vi "main.vi"() -> ()   [LabVIEW 2020]
doc: "该范例演示了通过VI查看其它VI的方法，还可运行和中止查看的VI。\n对于要中止的VI，应设置为可中止。对于无法中止的VI，可查看相关范例。"
uses:
  global/SettingVariable.vi
  global/GlobalVariable.vi
  utilities/TCPModbus_MasterClient.llb/MB Ethernet Master Query Read Input Registers (poly).vi
  utilities/TCPModbus_MasterClient.llb/MB Ethernet Master Query Write Multiple Registers (poly).vi
  <vilib>/Utility/config.llb/Write Key (Path).vi
  <vilib>/Utility/config.llb/NI_LVConfig.lvlib
panel:
  in  "退出":bool
  in  "Measure Square":bool
  in  "Physics Parameters Square":bool
  in  "Open Square":bool
  in  "Home Square":bool
  out "时间":string
  out "日期":string
  in  "MainPanel":enum32{"logo"}(tab)
  out "P2_8":dbl
  out "P2_7":dbl
  out "P2_6":dbl
  out "P2_5":dbl
  out "P2_4":dbl
  out "P2_3":dbl
  out "P2_2":dbl
  out "P2_1":dbl
  out "电流 2":dbl(slide)=1.0 scale=1e-13..0.0001 scale format="%#_2e"
  out "电流 1":dbl(slide)=1.0 scale=1e-13..0.0001 scale format="%#_2e"
  out "电压8":dbl(knob) caption="Gauge" scale=1.0..5.0
  out "电压7":dbl(knob)=1.0 caption="Gauge" scale=1.0..5.0
  out "电压6":dbl(knob)=1.0 caption="Gauge" scale=1.0..5.0
  out "电压5":dbl(knob)=1.0 caption="Gauge" scale=1.0..5.0
  out "电压4":dbl(knob)=1.0 caption="Gauge" scale=1.0..5.0
  out "电压3":dbl(knob)=1.0 caption="Gauge" scale=1.0..5.0
  out "电压2":dbl(knob) caption="Gauge" scale=1.0..5.0
  out "电压1":dbl(knob) caption="Gauge" scale=1.0..5.0
  in  "网络链接":bool
  # "iRho-100型反应性仪"
  # "Network"
  # "Current1"
  # "Current2"
  # "Voltage Output"
  # "Voltage Input"
  # "AC220V/50Hz"
  # "Ground"
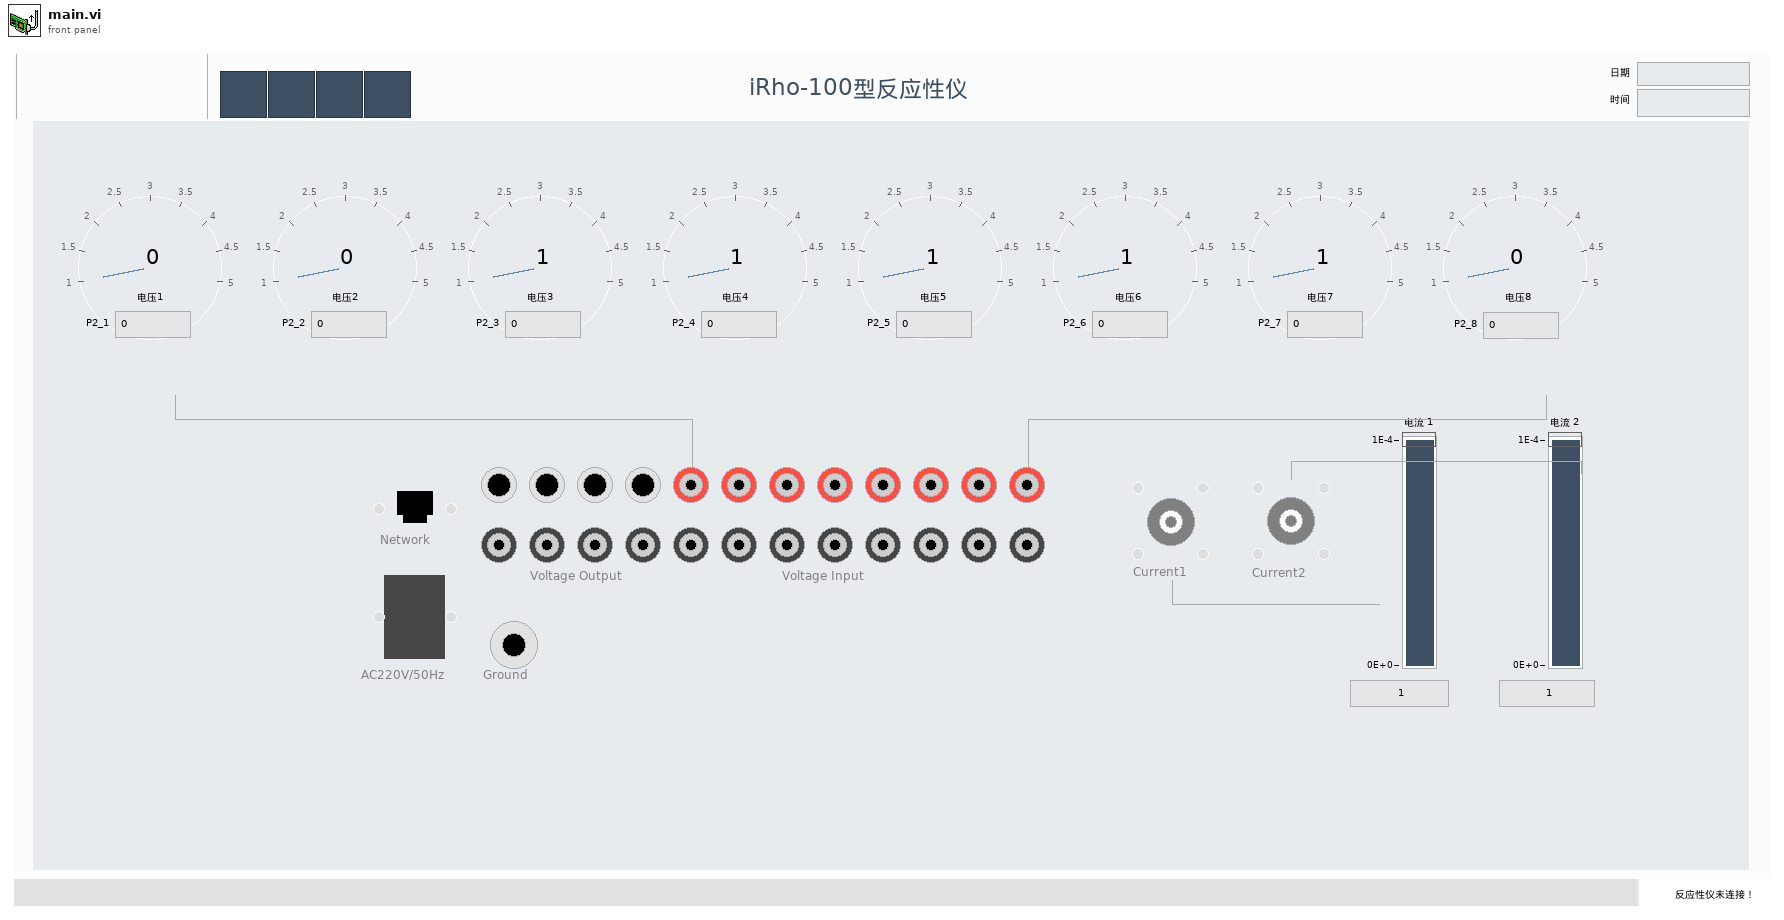
[diagram p1: front panel]
types:
  T1 = enum8{"Enabled", "Disabled", "Disabled and Grayed Out"}
  T2 = enum32{"Invalid", "Standard", "Closed", "Hidden", "Minimized", "Maximized"}
  T3 = cluster{"switch":bool, "name":string, "voltage upper":i32, "voltage lower":i32, "physics upper":dbl, "physics lower":dbl, "scale":u16}[]
  T4 = typedef "NI_LVConfig.lvlib/Config Data RefNum.ctl" = refnum<k1>
  T5 = enum32{"invalid app kind", "Development System", "Run Time System", "Student Edition", "Embedded LabVIEW", "Evaluation", "Custom"}
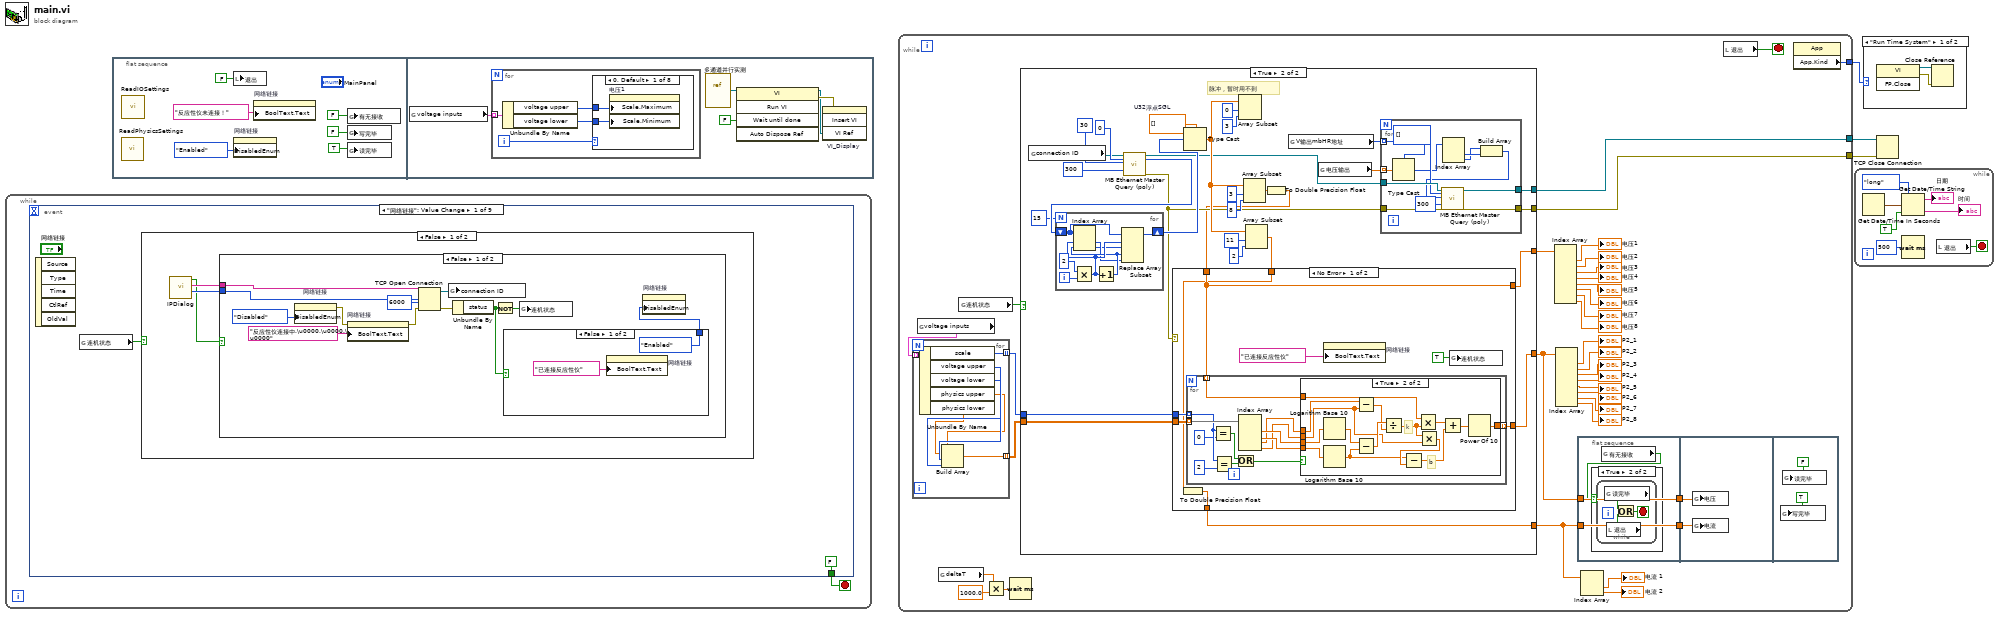
[diagram p0: block diagram]
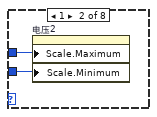
[diagram p2: hidden frame]
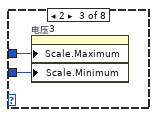
[diagram p3: hidden frame]
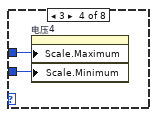
[diagram p4: hidden frame]
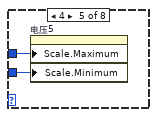
[diagram p5: hidden frame]
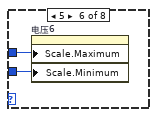
[diagram p6: hidden frame]
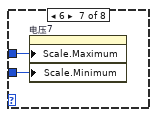
[diagram p7: hidden frame]
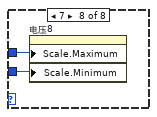
[diagram p8: hidden frame]
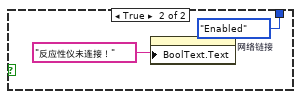
[diagram p9: hidden frame]
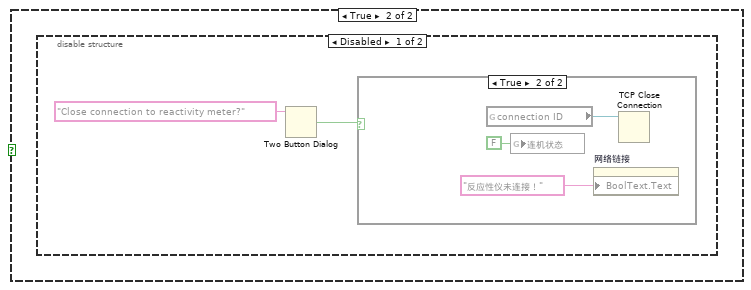
[diagram p11: hidden frame]
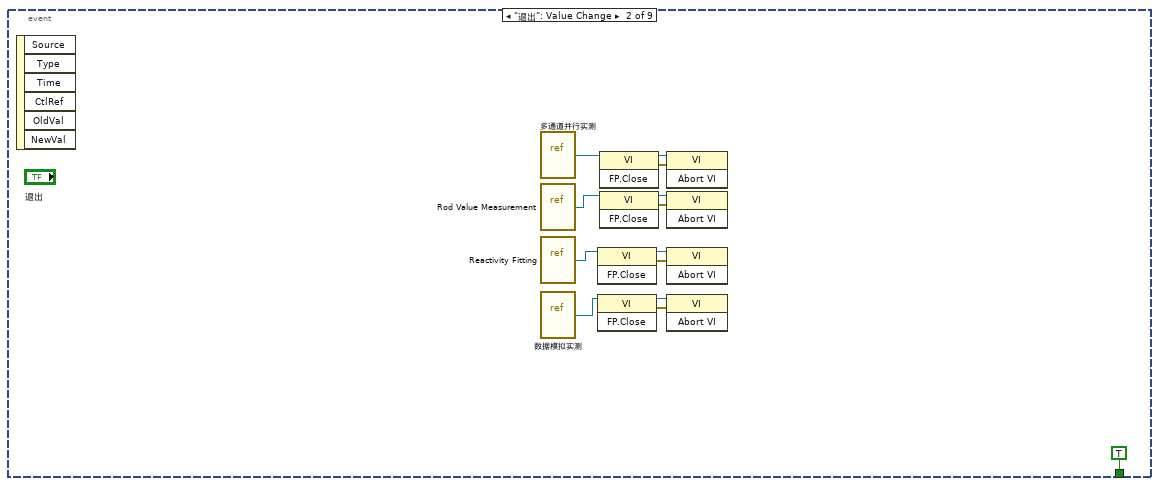
[diagram p14: hidden frame]
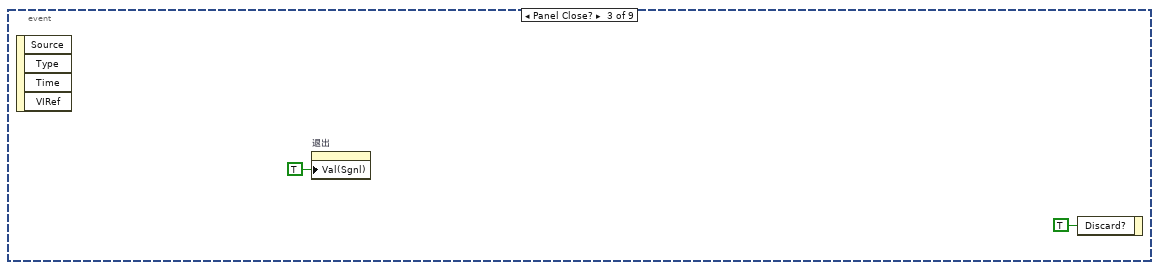
[diagram p15: hidden frame]
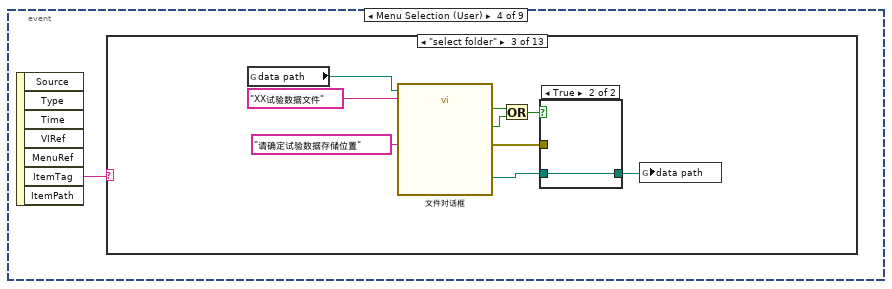
[diagram p16: hidden frame]
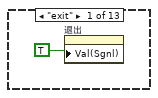
[diagram p17: hidden frame]
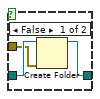
[diagram p19: hidden frame]
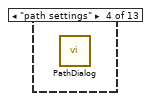
[diagram p20: hidden frame]
diagram:
  n1 = while {
    stop <- w4 stop-if-true
    n2 = event shown="[0] \"网络链接\": Value Change" {
      selector: _ -> [_ _ _ _ _ _ _ _ _]
      dyn-events: _ -> [_ _ _ _ _ _ _ _ _]
      timeout: _ -> [_ _ _ _ _ _ _ _ _]
      tunnel: [FALSE TRUE _ _ _ _ _ _ _] -> w4
      event "网络链接": Value Change {
        n3 = event-data() -> ()  [unwired: 1 in, 5 out]
        n4 = global read "GlobalVariable.vi" "连机状态"() -> (w5:bool)
        n5 = case shown="False" w5 {
          frame False {
            n6 = call "IPDialog.vi"() -> ("port"=w9:u16, "IP"=w8:string, "Cancelled?"=w7:bool)  [unwired: 9 in]
            n7 = case shown="False" w7 {
              tunnel: w9 -> [w12 _]
              tunnel: w8 -> [w11 _]
              frame False {
                n8 = property on="网络链接" class="Bool"("DisabledEnum"=T1."Disabled" ("Disabled")) -> (error out=w15:errorcluster)  [unwired: 2 in, 1 out]
                n9 = property on="网络链接" class="Bool"(error in=w15, "BoolText.Text"="反应性仪连接中.\u0000.\u0000.\u0000") -> (error out=w18:errorcluster)  [unwired: 1 in, 1 out]
                n10 = TCP Open Connection(address=w11, remote port or service name=w12, timeout ms (60000)=6000, error in (no error)=w18) -> (connection ID=w17:refnum<k5>, error out=w13:errorcluster)  [unwired: 1 out]
                n11 = global write "GlobalVariable.vi" "connection ID"(w17) -> ()
                n12 = Unbundle By Name(w13) -> ("status"=w19:bool)
                n13 = Not(x=w19) -> (.not. x?=w20:bool)
                n14 = case shown="False" w19 {
                  tunnel: [T1."Enabled" ("Disabled") T1."Enabled" ("Disabled")] -> w10
                  frame False {
                    n15 = property on="网络链接" class="Bool"("BoolText.Text"="已连接反应性仪") -> ()  [unwired: 2 in, 2 out]
                  }
                  frame True {
                    n16 = property on="网络链接" class="Bool"("BoolText.Text"="反应性仪未连接！") -> ()  [unwired: 2 in, 2 out]
                  }
                }
                n17 = global write "GlobalVariable.vi" "连机状态"(w20) -> ()
                n18 = property on="网络链接" class="Bool"("DisabledEnum"=w10) -> ()  [unwired: 2 in, 2 out]
              }
              frame True {
              }
            }
          }
          frame True {
            n19 = disable-structure shown="Disabled" {
              frame Disabled {
                n20 = Two Button Dialog(message="Close connection to reactivity meter?") -> (T button?=w26:bool)  [unwired: 2 in]
                n21 = case shown="True" w26 {
                  frame False {
                  }
                  frame True {
                    n22 = global read "GlobalVariable.vi" "connection ID"() -> (w30:refnum<k5>)
                    n23 = global write "GlobalVariable.vi" "连机状态"(FALSE ("连机状态")) -> ()
                    n24 = property on="网络链接" class="Bool"("BoolText.Text"="反应性仪未连接！" ("Boolean Text.Text")) -> ()  [unwired: 2 in, 2 out]
                    n25 = TCP Close Connection ("关闭TCP连接")(connection ID=w30) -> ()  [unwired: 1 in, 3 out]
                  }
                }
              }
              frame Enabled {
              }
            }
          }
        }
      }
      event "退出": Value Change {
        n26 = event-data() -> ()  [unwired: 1 in, 6 out]
        n27 = vi-ref "多通道并行实测.vi"() -> (w42:refnum<vi>)
        n28 = vi-ref "Rod Value Measurement.vi"() -> (w41:refnum<vi>)
        n29 = vi-ref "Reactivity Fitting.vi"() -> (w39:refnum<vi>)
        n30 = vi-ref "数据模拟实测.vi"() -> (w40:refnum<vi>)
        n31 = invoke class="VI" method="FP.Close"(reference=w39) -> (reference out=w34:refnum<vi>, error out=w33:errorcluster)  [unwired: 2 in, 1 out]
        n32 = invoke class="VI" method="FP.Close"(reference=w40) -> (reference out=w32:refnum<vi>, error out=w31:errorcluster)  [unwired: 2 in, 1 out]
        n33 = invoke class="VI" method="FP.Close"(reference=w42) -> (reference out=w38:refnum<vi>, error out=w37:errorcluster)  [unwired: 2 in, 1 out]
        n34 = invoke class="VI" method="FP.Close"(reference=w41) -> (reference out=w36:refnum<vi>, error out=w35:errorcluster)  [unwired: 2 in, 1 out]
        n35 = invoke class="VI" method="Abort VI"(reference=w38, error in=w37) -> ()  [unwired: 1 in, 3 out]
        n36 = invoke class="VI" method="Abort VI"(reference=w36, error in=w35) -> ()  [unwired: 1 in, 3 out]
        n37 = invoke class="VI" method="Abort VI"(reference=w34, error in=w33) -> ()  [unwired: 1 in, 3 out]
        n38 = invoke class="VI" method="Abort VI"(reference=w32, error in=w31) -> ()  [unwired: 1 in, 3 out]
      }
      event Panel Close? {
        n39 = event-data() -> ()  [unwired: 1 in, 4 out]
        n40 = property on="退出" class="Bool (strict)"("Val(Sgnl)"=TRUE ("Value (Signaling)")) -> ()  [unwired: 2 in, 2 out]
        n41 = event-data("Discard?"=TRUE) -> ()  [unwired: 1 in, 1 out]
      }
      event Menu Selection (User) {
        n42 = event-data() -> ("ItemTag"=w46:string)  [unwired: 1 in, 6 out]
        n43 = case shown="\"select folder\"" w46 {
          frame "exit" {
            n44 = property on="退出" class="Bool (strict)"("Val(Sgnl)"=TRUE) -> ()  [unwired: 2 in, 2 out]
          }
          frame Default {
          }
          frame "select folder" {
            n45 = global read "SettingVariable.vi" "data path"() -> (w49:path)
            n46 = call "文件对话框"("start path"=w49, "prompt"="请确定试验数据存储位置", "default name"="XX试验数据文件") -> ("selected path"=w56:path, "exists"=w54:bool, "cancelled"=w52:bool, "error out"=w55:errorcluster)  [unwired: 9 in]
            n47 = Or(x=w54, y=w52) -> (x .or. y?=w53:bool)
            n48 = case shown="True" w53 {
              tunnel: w56 -> [w59 w60]
              tunnel: w55 -> [w58 _]
              tunnel: [w57 w60] -> w48
              frame False {
                n49 = Create Folder(path (use dialog)=w59, error in=w58) -> (created path=w57:path)  [unwired: 1 in, 2 out]
              }
              frame True {
              }
            }
            n50 = global write "SettingVariable.vi" "data path"(w48) -> ()
          }
          frame "path settings" {
            n51 = call "PathDialog.vi"() -> ()  [unwired: 11 in, 1 out]
          }
          frame "physics settings" {
            n52 = call "PhysicsDialog.vi"() -> ()  [unwired: 1 in]
          }
          frame "input settings" {
            n53 = call "InputDialog.vi"() -> ("Cancelled?"=w61:bool)  [unwired: 9 in]
            n54 = case shown="True" w61 {
              frame False {
              }
              frame True {
                n55 = global read "SettingVariable.vi" "voltage inputs"() -> (w62:T3)
                n56 = for {
                  tunnel: w62 -> [w66] mode=indexing
                  i -> [w65]
                  n57 = Unbundle By Name(w66) -> ("voltage upper"=w64:i32, "voltage lower"=w63:i32)
                  n58 = case shown="0, Default" w65 {
                    tunnel: w64 -> [w68 w70 w72 w74 w76 w78 w80 w82]
                    tunnel: w63 -> [w67 w69 w71 w73 w75 w77 w79 w81]
                    frame 0, Default {
                      n59 = property on="电压1" class="Knob (strict)"("Scale.Maximum"=w68, "Scale.Minimum"=w67) -> ()  [unwired: 2 in, 2 out]
                    }
                    frame 1 {
                      n60 = property on="电压2" class="Knob (strict)"("Scale.Maximum"=w70, "Scale.Minimum"=w69) -> ()  [unwired: 2 in, 2 out]
                    }
                    frame 2 {
                      n61 = property on="电压3" class="Knob (strict)"("Scale.Maximum"=w72, "Scale.Minimum"=w71) -> ()  [unwired: 2 in, 2 out]
                    }
                    frame 3 {
                      n62 = property on="电压4" class="Knob (strict)"("Scale.Maximum"=w74, "Scale.Minimum"=w73) -> ()  [unwired: 2 in, 2 out]
                    }
                    frame 4 {
                      n63 = property on="电压5" class="Knob (strict)"("Scale.Maximum"=w76, "Scale.Minimum"=w75) -> ()  [unwired: 2 in, 2 out]
                    }
                    frame 5 {
                      n64 = property on="电压6" class="Knob (strict)"("Scale.Maximum"=w78, "Scale.Minimum"=w77) -> ()  [unwired: 2 in, 2 out]
                    }
                    frame 6 {
                      n65 = property on="电压7" class="Knob (strict)"("Scale.Maximum"=w80, "Scale.Minimum"=w79) -> ()  [unwired: 2 in, 2 out]
                    }
                    frame 7 {
                      n66 = property on="电压8" class="Knob (strict)"("Scale.Maximum"=w82, "Scale.Minimum"=w81) -> ()  [unwired: 2 in, 2 out]
                    }
                  }
                }
              }
            }
          }
          frame "output settings" {
            n67 = call "OutputDialog.vi"() -> ()  [unwired: 11 in, 1 out]
          }
          frame "homepage" {
            n68 = property on="VI_Display" class="SubPnl"("Visible"=FALSE) -> ()  [unwired: 2 in, 2 out]
          }
          frame "monitor" {
            n69 = property on="VI_Display" class="SubPnl"("Visible"=TRUE) -> ()  [unwired: 2 in, 2 out]
          }
          frame "rod measurement" {
            n70 = vi-ref "Rod Value Measurement.vi"() -> (w87:refnum<vi>)
            n71 = invoke class="VI" method="FP.Open"(reference=w87, "Activate"=TRUE ("Activate?"), "State"=T2."Standard") -> (reference out=w88:refnum<vi>)  [unwired: 2 in, 4 out]
            n72 = invoke class="VI" method="Run VI"(reference=w88, "Wait until done"=FALSE ("Wait Until Done"), "Auto Dispose Ref"=FALSE ("Auto Dispose Reference")) -> ()  [unwired: 2 in, 5 out]
          }
          frame "reactivity fitting" {
            n73 = vi-ref "Reactivity Fitting.vi"() -> (w93:refnum<vi>)
            n74 = invoke class="VI" method="FP.Open"(reference=w93, "Activate"=TRUE ("Activate?"), "State"=T2."Standard") -> (reference out=w94:refnum<vi>)  [unwired: 2 in, 4 out]
            n75 = invoke class="VI" method="Run VI"(reference=w94, "Wait until done"=FALSE ("Wait Until Done"), "Auto Dispose Ref"=FALSE ("Auto Dispose Reference")) -> ()  [unwired: 2 in, 5 out]
          }
          frame "history simulation" {
            n76 = vi-ref "数据模拟实测.vi"() -> (w99:refnum<vi>)
            n77 = invoke class="VI" method="FP.Open"(reference=w99, "Activate"=TRUE ("Activate?"), "State"=T2."Standard") -> (reference out=w100:refnum<vi>)  [unwired: 2 in, 4 out]
            n78 = invoke class="VI" method="Run VI"(reference=w100, "Wait until done"=FALSE ("Wait Until Done"), "Auto Dispose Ref"=FALSE ("Auto Dispose Reference")) -> ()  [unwired: 2 in, 5 out]
          }
          frame "about" {
            n79 = call "About.vi"() -> ()  [unwired: 1 in]
          }
        }
      }
      event "Home Square": Value Change {
        n80 = event-data() -> ()  [unwired: 1 in, 6 out]
        n81 = property on="VI_Display" class="SubPnl"("Visible"=FALSE) -> ()  [unwired: 2 in, 2 out]
      }
      event "Measure Square": Value Change {
        n82 = event-data() -> ()  [unwired: 1 in, 6 out]
        n83 = property on="VI_Display" class="SubPnl"("Visible"=TRUE) -> ()  [unwired: 2 in, 2 out]
      }
      event "Open Square": Value Change {
        n84 = event-data() -> ()  [unwired: 1 in, 6 out]
        n85 = global read "SettingVariable.vi" "data path"() -> (w105:path)
        n86 = call <vilib>:"Space Constant.vi"() -> ("String"=w119:string)
        n87 = Path To String(path=w105) -> (string=w116:string)
        n88 = Concatenate Strings("explorer" ("字符串"), w119, w116) -> (w117:string)
        n89 = call <vilib>:"System Exec.vi"("command line"=w117) -> ()  [unwired: 7 in, 4 out]
        n90 = call <vilib>:"Application Directory.vi"() -> ("Application Directory"=w111:path)
        n91 = Build Path(base path=w111, name or relative path=path "configure.ini") -> (appended path=w112:path)
        n92 = call <vilib>:"Open Config Data.vi"("configuration file path"=w112) -> ("error out"=w114:errorcluster, "refnum"=w113:T4)  [unwired: 2 in, 7 out]
        n93 = call-poly <vilib>:"Write Key.vi"("section"="Path", "error in (no error)"=w114, "value"=w105, "key"="data" ("section"), "refnum"=w113) -> ("error out"=w109:errorcluster, "refnum out"=w110:T4)  [unwired: 4 in, 1 out]
        n94 = call <vilib>:"Close Config Data.vi"("error in (no error)"=w109, "refnum"=w110) -> ("error out"=w115:errorcluster)  [unwired: 1 in, 8 out]
        n95 = call <vilib>:"Simple Error Handler.vi"("error in (no error)"=w115) -> ()  [unwired: 1 in, 8 out]
      }
      event "Physics Parameters Square": Value Change {
        n96 = event-data() -> ()  [unwired: 1 in, 6 out]
        n97 = call "PhysicsDialog.vi"() -> ()  [unwired: 1 in]
      }
      event "时间": Shortcut Menu Selection (User) {
        n98 = event-data() -> ("ItemTag"=w120:string)  [unwired: 1 in, 7 out]
        n99 = case shown="\"time calibration\", Default" w120 {
          frame "time calibration", Default {
            n100 = global read "GlobalVariable.vi" "连机状态"() -> (w121:bool)
            n101 = case shown="True" w121 {
              frame False {
                n102 = One Button Dialog(message="未连接反应性仪") -> ()  [unwired: 1 in, 1 out]
              }
              frame True {
                w129 = "%x" ("格式字符串")
                w130 = u16[] [] ("数组类型(2D Dbl)")
                n103 = Get Date/Time String(want seconds? (F)=TRUE ("需要秒？(F)")) -> (date string=w146:string, time string=w145:string)  [unwired: 2 in]
                n104 = Spreadsheet String To Array(delimiter (Tab)="/" ("分隔符(Tab)"), format string=w129, spreadsheet string=w146, array type (2D Dbl)=w130) -> (array=w142:u16[])
                n105 = Spreadsheet String To Array(delimiter (Tab)=":" ("分隔符(Tab)"), format string=w129, spreadsheet string=w145, array type (2D Dbl)=w130) -> (array=w140:u16[])
                n106 = Index Array(array=w142, index=0 ("索引")) -> (element=w144:u16)
                n107 = Subtract(x=w144, y=u16 8192) -> (x-y=w143:u16)
                n108 = Replace Array Subset(array=w142, new element=w143, index=0 ("索引")) -> (w141:u16[])
                n109 = Build Array (concatenate)(w141, w140) -> (w139:u16[])
                n110 = To Unsigned Byte Integer(number=w139) -> (unsigned 8bit integer=w138:u8[])
                n111 = for {
                  N: 3 -> [_]
                  shift-right: [w148] -> w137
                  shift-left: w138 -> [w153]
                  i -> [w155]
                  n112 = Multiply(x=2, y=w155) -> (x*y=w152:i32)
                  n113 = Increment(x=w152) -> (x+1=w151:i32)
                  n114 = Index Array(array=w153, index #1=w152, index #2=w151) -> (element #1=w150:u8, element #2=w149:u8)
                  n115 = Replace Array Subset(array=w153, new element #1=w149, index #1=w152, new element #2=w150, index #2=w151) -> (w148:u8[])
                }
                n116 = global read "GlobalVariable.vi" "connection ID"() -> (w123:refnum<k5>)
                n117 = Type Cast(type=u16[] [] ("Input Registers"), x=w137) -> (*(type *) &x=w125:u16[])
                n118 = call-poly "MB Ethernet Master Query (poly).vi"("TCP Connection Refnum in"=w123, "Starting Address"=u16 65436, "Registers"=w125) -> ("error out"=w124:errorcluster)  [unwired: 3 in, 13 out]
                n119 = case shown="Error .." w124 {
                  frame No Error {
                  }
                  frame Error {
                    n120 = One Button Dialog(message="写入失败！请检查网络连接。") -> ()  [unwired: 1 in, 1 out]
                  }
                }
              }
            }
          }
        }
      }
    }
  }
  n121 = flat-sequence {
    frame #0 {
      n122 = call "ReadPhysicsSettings.vi"() -> ()  [unwired: 12 in]
      n123 = call "ReadIOSettings.vi"() -> ()  [unwired: 12 in]
      n124 = local write "退出"(FALSE ("退出")) -> ()
      n125 = property on="网络链接" class="Bool"("DisabledEnum"=T1."Enabled" ("Disabled")) -> ()  [unwired: 2 in, 2 out]
      n126 = property on="网络链接" class="Bool"("BoolText.Text"="反应性仪未连接！") -> ()  [unwired: 2 in, 2 out]
      n127 = global write "GlobalVariable.vi" "有无接收"(FALSE ("读完毕")) -> ()
      n128 = global write "GlobalVariable.vi" "写完毕"(FALSE ("读完毕")) -> ()
      n129 = global write "GlobalVariable.vi" "读完毕"(TRUE ("读完毕")) -> ()
    }
    frame #1 {
      n130 = global read "SettingVariable.vi" "voltage inputs"() -> (w166:T3)
      n131 = for {
        tunnel: w166 -> [w170] mode=indexing
        i -> [w169]
        n132 = Unbundle By Name(w170) -> ("voltage upper"=w168:i32, "voltage lower"=w167:i32)
        n133 = case shown="0, Default" w169 {
          tunnel: w168 -> [w172 w174 w176 w178 w180 w182 w184 w186]
          tunnel: w167 -> [w171 w173 w175 w177 w179 w181 w183 w185]
          frame 0, Default {
            n134 = property on="电压1" class="Knob (strict)"("Scale.Maximum"=w172, "Scale.Minimum"=w171) -> ()  [unwired: 2 in, 2 out]
          }
          frame 1 {
            n135 = property on="电压2" class="Knob (strict)"("Scale.Maximum"=w174, "Scale.Minimum"=w173) -> ()  [unwired: 2 in, 2 out]
          }
          frame 2 {
            n136 = property on="电压3" class="Knob (strict)"("Scale.Maximum"=w176, "Scale.Minimum"=w175) -> ()  [unwired: 2 in, 2 out]
          }
          frame 3 {
            n137 = property on="电压4" class="Knob (strict)"("Scale.Maximum"=w178, "Scale.Minimum"=w177) -> ()  [unwired: 2 in, 2 out]
          }
          frame 4 {
            n138 = property on="电压5" class="Knob (strict)"("Scale.Maximum"=w180, "Scale.Minimum"=w179) -> ()  [unwired: 2 in, 2 out]
          }
          frame 5 {
            n139 = property on="电压6" class="Knob (strict)"("Scale.Maximum"=w182, "Scale.Minimum"=w181) -> ()  [unwired: 2 in, 2 out]
          }
          frame 6 {
            n140 = property on="电压7" class="Knob (strict)"("Scale.Maximum"=w184, "Scale.Minimum"=w183) -> ()  [unwired: 2 in, 2 out]
          }
          frame 7 {
            n141 = property on="电压8" class="Knob (strict)"("Scale.Maximum"=w186, "Scale.Minimum"=w185) -> ()  [unwired: 2 in, 2 out]
          }
        }
      }
      n142 = vi-ref "多通道并行实测.vi"() -> (w163:refnum<vi>)
      n143 = invoke class="VI" method="Run VI"(reference=w163, "Wait until done"=FALSE ("Wait Until Done")) -> (reference out=w164:refnum<vi>, error out=w165:errorcluster)  [unwired: 3 in, 3 out]
      n144 = invoke on="VI_Display" class="SubPnl" method="Insert VI"(error in=w165, "VI Ref"=w164) -> ()  [unwired: 2 in, 4 out]
    }
  }
  n145 = while {
    tunnel: [w193] -> w2
    tunnel: [w192] -> w1
    tunnel: [w195] -> w3
    stop <- w194 stop-if-true
    n146 = global read "SettingVariable.vi" "voltage inputs"() -> (w190:T3)
    n147 = for {
      tunnel: w190 -> [w227] mode=indexing
      tunnel: [w226] -> w189 mode=indexing
      tunnel: [w221] -> w188 mode=indexing
      n148 = Unbundle By Name(w227) -> ("scale"=w226:u16, "voltage upper"=w225:i32, "voltage lower"=w224:i32, "physics upper"=w223:dbl, "physics lower"=w222:dbl)
      n149 = Build Array(w223, w222, w225, w224) -> (w221:dbl[])
    }
    n150 = global read "SettingVariable.vi" "deltaT"() -> (w191:dbl)
    n151 = global read "GlobalVariable.vi" "连机状态"() -> (w187:bool)
    n152 = Multiply(x=w191, y=1000.0) -> (x*y=w197:dbl)
    n153 = Wait (ms)(milliseconds to wait=w197) -> ()  [unwired: 1 out]
    n154 = case shown="True" w187 {
      tunnel: w189 -> [_ w237]
      tunnel: w188 -> [_ w238]
      tunnel: [dbl[] [nan, nan, nan, nan, nan, nan, nan, nan] w236] -> w218
      tunnel: [dbl[] [nan, nan] w233] -> w217
      tunnel: [dbl[] [nan, nan, nan, nan, nan, nan, nan, nan] w239] -> w196
      tunnel: [w232 w242] -> w193
      tunnel: [errorcluster {"status"=FALSE, "code"=0, "source"=""} ("error out") w241] -> w192
      frame False {
        n155 = global read "GlobalVariable.vi" "connection ID"() -> (w232:refnum<k5>)
      }
      frame True {
        w250 = sgl[] []  # U32浮点SGL
        # "脉冲，暂时用不到"
        n156 = global read "GlobalVariable.vi" "connection ID"() -> (w244:refnum<k5>)
        n157 = call-poly "MB Ethernet Master Query (poly).vi"("TCP Connection Refnum in"=w244, "Starting Address"=u16 0, "Quantity"=u16 30 ("modbus寄存器数量"), "Timeout"=300) -> ("TCP Connection Refnum (dup)"=w243:refnum<k5>, "Input Registers"=w248:u16[], "error out"=w240:errorcluster)  [unwired: 1 in, 12 out]
        n158 = for {
          N: 15 -> [_]
          shift-right: [w262] -> w247
          shift-left: w248 -> [w267]
          i -> [w269]
          n159 = Multiply(x=2, y=w269) -> (x*y=w266:i32)
          n160 = Increment(x=w266) -> (x+1=w265:i32)
          n161 = Index Array(array=w267, index #1=w266, index #2=w265) -> (element #1=w264:u16, element #2=w263:u16)
          n162 = Replace Array Subset(array=w267, new element #1=w263, index #1=w266, new element #2=w264, index #2=w265) -> (w262:u16[])
        }
        n163 = Type Cast(type=w250, x=w247) -> (*(type *) &x=w254:sgl[])
        n164 = Array Subset(array=w254, index=0 ("索引"), length=3 ("长度")) -> ()  [unwired: 1 out]
        n165 = Array Subset(array=w254, index=3 ("索引"), length=8 ("长度")) -> (w257:sgl[])
        n166 = Array Subset(array=w254, index=11 ("索引"), length=2 ("长度")) -> (w234:sgl[])
        n167 = To Double Precision Float(number=w257) -> (double precision float=w235:dbl[])
        n168 = case shown="No Error" w240 {
          tunnel: [w289 dbl[] [nan, nan, nan, nan, nan, nan, nan, nan]] -> w239
          tunnel: w235 -> [w289 _]
          tunnel: w238 -> [w288 _]
          tunnel: w237 -> [w287 _]
          tunnel: [w286 dbl[] [nan, nan, nan, nan, nan, nan, nan, nan]] -> w236
          tunnel: w234 -> [w283 _]
          tunnel: [w282 dbl[] [nan, nan]] -> w233
          frame No Error {
            n169 = To Double Precision Float(number=w283) -> (double precision float=w282:dbl[])
            n170 = for {
              tunnel: w289 -> [w301] mode=indexing
              tunnel: [w300] -> w286 mode=indexing
              tunnel: w288 -> [w302] mode=indexing
              tunnel: w287 -> [w299] mode=indexing
              n171 = Equal?(x=w299, y=u16 0) -> (x = y?=w296:bool)
              n172 = Equal?(x=w299, y=u16 2) -> (x = y?=w295:bool)
              n173 = Or(x=w296, y=w295) -> (x .or. y?=w294:bool)
              n174 = Index Array(array=w302) -> (element #1=w293:dbl, element #2=w292:dbl, element #3=w291:dbl, element #4=w290:dbl)  [unwired: 4 in]
              n175 = case shown="True" w294 {
                tunnel: w301 -> [w314 w320]
                tunnel: [w313 w318] -> w300
                tunnel: w291 -> [w306 w323]
                tunnel: w290 -> [w305 w322]
                tunnel: w293 -> [w304 w316]
                tunnel: w292 -> [w303 w321]
                frame False {
                  # "b"
                  # "k"
                  n176 = Subtract(x=w306, y=w305) -> (x-y=w311:dbl)
                  n177 = Subtract(x=w304, y=w303) -> (x-y=w312:dbl)
                  n178 = Divide(x=w312, y=w311) -> (x/y=w310:dbl)
                  n179 = Multiply(x=w314, y=w310) -> (x*y=w308:dbl)
                  n180 = Multiply(x=w310, y=w305) -> (x*y=w309:dbl)
                  n181 = Subtract(x=w303, y=w309) -> (x-y=w307:dbl)
                  n182 = Add(x=w308, y=w307) -> (x+y=w313:dbl)
                }
                frame True {
                  # "b"
                  # "k"
                  n183 = Logarithm Base 10(1:w316) -> (0:w315:dbl)
                  n184 = Logarithm Base 10(1:w321) -> (0:w317:dbl)
                  n185 = Subtract(x=w323, y=w322) -> (x-y=w328:dbl)
                  n186 = Subtract(x=w315, y=w317) -> (x-y=w329:dbl)
                  n187 = Divide(x=w329, y=w328) -> (x/y=w327:dbl)
                  n188 = Multiply(x=w320, y=w327) -> (x*y=w325:dbl)
                  n189 = Multiply(x=w327, y=w322) -> (x*y=w326:dbl)
                  n190 = Subtract(x=w317, y=w326) -> (x-y=w324:dbl)
                  n191 = Add(x=w325, y=w324) -> (x+y=w319:dbl)
                  n192 = Power Of 10(x=w319) -> (10^x=w318:dbl)
                }
              }
            }
            n193 = property on="网络链接" class="Bool"("BoolText.Text"="已连接反应性仪") -> ()  [unwired: 2 in, 2 out]
            n194 = global write "GlobalVariable.vi" "连机状态"(TRUE ("连机状态")) -> ()
          }
          frame Error {
            n195 = property on="网络链接" class="Bool"("BoolText.Text"="反应性仪未连接！") -> ()  [unwired: 2 in, 2 out]
            n196 = global write "GlobalVariable.vi" "连机状态"(FALSE ("连机状态")) -> ()
          }
        }
        n197 = global read "GlobalVariable.vi" "V输出mbHR地址"() -> (w252:u16[])
        n198 = global read "GlobalVariable.vi" "电压输出"() -> (w253:sgl[])
        n199 = for {
          tunnel: w240 -> [w281]
          tunnel: w243 -> [w280]
          tunnel: [w279] -> w241
          tunnel: [w278] -> w242
          tunnel: w253 -> [w277] mode=indexing
          tunnel: w252 -> [w276] mode=indexing
          n200 = Type Cast(type=u16[] [] ("Input Registers"), x=w277) -> (*(type *) &x=w274:u16[])
          n201 = Index Array(array=w274) -> (element #1=w273:u16, element #2=w272:u16)  [unwired: 2 in]
          n202 = Build Array(w272, w273) -> (w271:u16[])
          n203 = call-poly "MB Ethernet Master Query (poly).vi"("TCP Connection Refnum in"=w280, "Starting Address"=w276, "Registers"=w271, "Timeout"=u32 300, "error in"=w281) -> ("TCP Connection Refnum (dup)"=w278:refnum<k5>, "error out"=w279:errorcluster)  [unwired: 1 in, 12 out]
        }
      }
    }
    n204 = Index Array(array=w196) -> (element #1=→"电压1":dbl, element #2=→"电压2":dbl, element #3=→"电压3":dbl, element #4=→"电压4":dbl, element #5=→"电压5":dbl, element #6=→"电压6":dbl, element #7=→"电压7":dbl, element #8=→"电压8":dbl)  [unwired: 8 in]
    n205 = Index Array(array=w218) -> (element #1=→"P2_1":dbl, element #2=→"P2_2":dbl, element #3=→"P2_3":dbl, element #4=→"P2_4":dbl, element #5=→"P2_5":dbl, element #6=→"P2_6":dbl, element #7=→"P2_7":dbl, element #8=→"P2_8":dbl)  [unwired: 8 in]
    n206 = flat-sequence {
      tunnel: w217 -> [w336]
      tunnel: w218 -> [w337]
      tunnel: [w337] -> w220
      tunnel: [w336] -> w219
      tunnel: w220 -> [w342]
      tunnel: w219 -> [w341]
      frame #0 {
        n207 = global read "GlobalVariable.vi" "有无接收"() -> (w335:bool)
        n208 = case shown="True" w335 {
          frame False {
          }
          frame True {
            n209 = while {
              stop <- w339 stop-if-true
              n210 = global read "GlobalVariable.vi" "读完毕"() -> (w338:bool)
              n211 = local read "退出"() -> (w340:bool)
              n212 = Or(x=w338, y=w340) -> (x .or. y?=w339:bool)
            }
          }
        }
      }
      frame #1 {
        n213 = global write "GlobalVariable.vi" "电压"(w342) -> ()
        n214 = global write "GlobalVariable.vi" "电流"(w341) -> ()
      }
      frame #2 {
        n215 = global write "GlobalVariable.vi" "写完毕"(TRUE ("写完毕")) -> ()
        n216 = global write "GlobalVariable.vi" "读完毕"(FALSE ("写完毕")) -> ()
      }
    }
    n217 = Index Array(array=w217) -> (element #1=→"电流 1":dbl, element #2=→"电流 2":dbl)  [unwired: 2 in]
    n218 = local read "退出"() -> (w194:bool)
    n219 = property class="App"() -> ("App.Kind"=w195:T5)  [unwired: 2 in, 2 out]
  }
  n220 = while {
    stop <- w347 stop-if-true
    n221 = Get Date/Time In Seconds() -> (seconds since 1Jan1904=w351:timestamp)
    n222 = Get Date/Time String(date format (0)=enum16{"short", "long", "abbreviated"}."long" ("日期格式(0)"), seconds (now)=w351, want seconds? (F)=TRUE) -> (date string=→"日期":string, time string=→"时间":string)
    n223 = Wait (ms)(milliseconds to wait=u32 500) -> ()  [unwired: 1 out]
    n224 = local read "退出"() -> (w347:bool)
  }
  n225 = case shown="\"Run Time System\"" w3 {
    frame "Run Time System" {
      n226 = invoke class="VI" method="FP.Close"() -> (reference out=w352:refnum<vi>, error out=w353:errorcluster)  [unwired: 3 in, 1 out]
      n227 = Close Reference(reference=w352, error in (no error)=w353) -> ()  [unwired: 1 out]
    }
    frame "Development System", Default {
    }
  }
  n228 = TCP Close Connection ("关闭TCP连接")(connection ID=w2, error in (no error)=w1) -> ()  [unwired: 3 out]
